vi "pid-toolkit-autotuning-design.vi"() -> ()   [LabVIEW 2018, in "pid-toolkit.lvlib"]
uses:
  <vilib>/Platform/TimedLoop/XDataNode/timing_clust.ctl
  <vilib>/Platform/TimedLoop/XDataNode/nitl_modes.ctl
  <vilib>/Platform/TimedLoop/XDataNode/wakeup.ctl
  <vilib>/addons/control/pid/autopid.llb/PID Autotuning Design (Ziegler-Nichols).vi
  <vilib>/addons/control/pid/autopid.llb/PID Autotuning Design (Cohen-Coon).vi
  <vilib>/addons/control/pid/autopid.llb/PID Autotuning Design (Chien-Hrones-Reswick).vi
  <vilib>/addons/control/pid/autopid.llb/PID Autotuning Design (Internal Model Control).vi
  <vilib>/platform/TimedLoop/XDataNode/XDataNode.xnode
  pid-toolkit.lvlib
  <vilib>/Platform/TimedLoop/XDataNode/XDNodeRunTimeDep.lvlib
  <vilib>/addons/control/pid/NI_PID_autopid.lvlib
panel:
  in  "Tuning specifications":u16(ring) items=["Regulator - 0 %", "Regulator -  20%", "Servo - 0%", "Servo - 20%"]
  in  "Desired Time Constant (tau_c)":dbl
  out "Single Update (Multiple Plots, stacked)":cluster{"Temperature":sgl, "Setpoint":sgl, sgl}(graph)
  out "Output":u16
  out "High":bool
  out "Low":bool
  in  "Manual":u8(slide) scale=0.0..255.0
  out "Stimulus":dbl
  out "Response":dbl
  out "Plant Parameters":T1
  out "PID gains":T2
  in  "Controller Gain (K)":dbl
  in  "Closed Loop":bool
  in  "Ziegler-Nichols Speed":u16(ring) items=["Fast", "Normal", "Slow"]
  out "size(s)":i32
  in  "Method":T3(ring)
  in  "Type of Controller":u16(ring) items=["P", "PI", "PID"]
  out "Modbus error":errorcluster
  in  "Off Hook":bool
  in  "Update Rate":dbl caption="Rate"
  out "Failure":bool
  out "Updating":bool
  in  "Update Now":bool
  in  "Maximum":sgl
  in  "Minimum":sgl
  out "Thermometer":sgl(slide) scale=0.0..260.0
  in  "Force exit out of loop":bool
  out "Interval":i64
  out "Duration":i64
  out "Cycle":i32
  in  "Frequency":dbl(slide) scale=0.1..10.0
  # "Loop"
  # "Modbus"
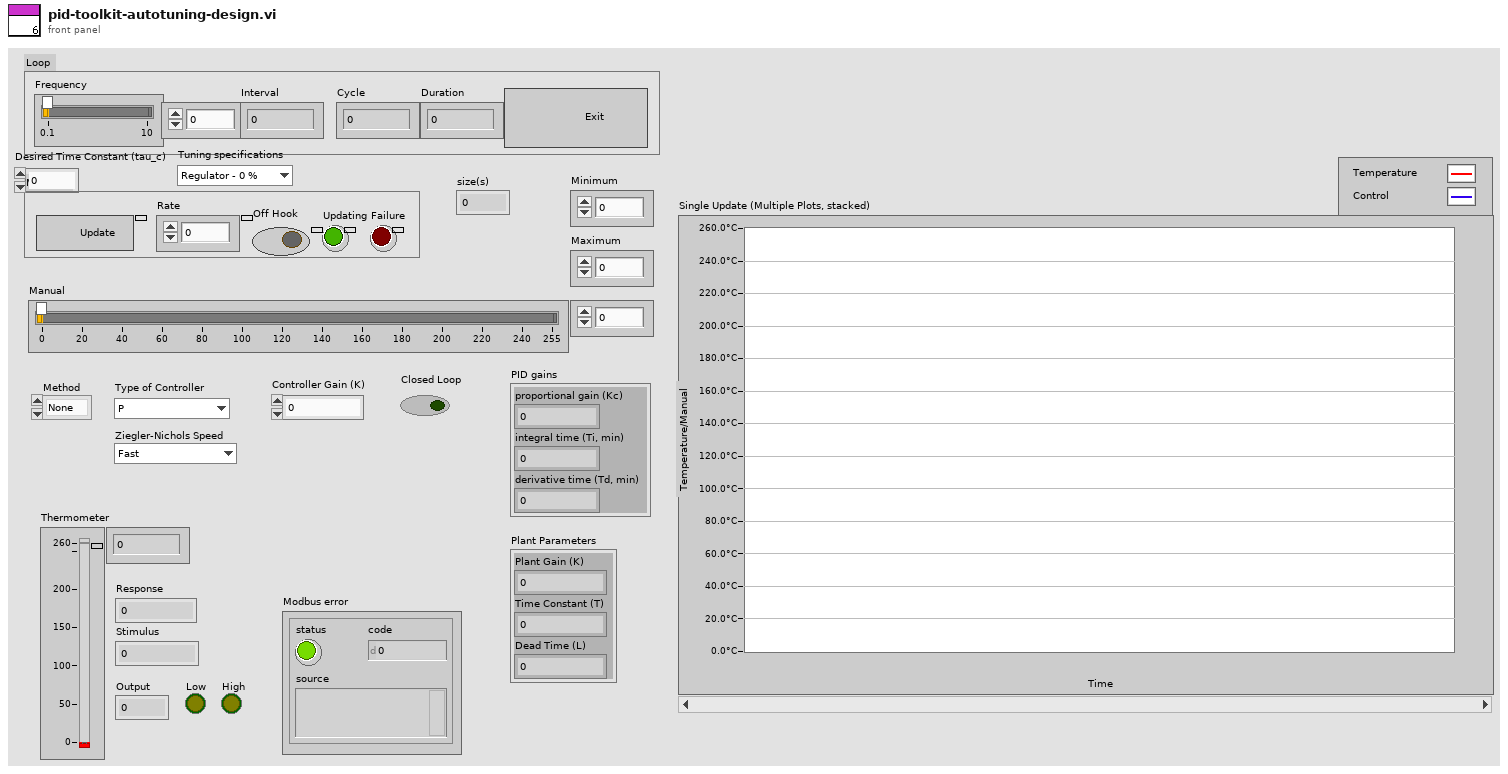
[diagram p1: front panel]
types:
  T1 = cluster{"Plant Gain (K)":dbl, "Time Constant (T)":dbl, "Dead Time (L)":dbl}
  T2 = cluster{"proportional gain (Kc)":dbl, "integral time (Ti, min)":dbl, "derivative time (Td, min)":dbl}
  T3 = enum16{"None", "Ziegler-Nichols", "Cohen-Coon", "Chien-Hrones-Reswick", "Internal Model Control"}
  T4 = typedef "XDNodeRunTimeDep.lvlib/timing_clust.ctl" = cluster{"Expected End [f-1]":u64, "Actual End [f-1]":u64, "Finished Late? [f-1]":bool, "Expected End [i-1]":u64, "Actual End [i-1]":u64, "Finished Late? [i-1]":bool, "Expected Start [i]":u64, "Actual Start [i]":u64, "Expected Start [f]":u64, "Actual Start [f]":u64, "Source Name":string, "Structure Name":string, "Period":i64, "Deadline":i64, "Offset":i64, "Start":i64, "Priority":i32, "Timeout":i32, "Mode":T5, "Wakeup Reason":T6, "Error":errorcluster, "Source Type":string, "Secondary Source Type":string, "Global End Time":u64, "Global Start Time":u64, "Frame Duration":u64, "Iteration Duration":u64, "Assigned CPU":i32, "I/O Scan Engine Mode":u32}
  T5 = typedef "XDNodeRunTimeDep.lvlib/nitl_modes.ctl" = enum32{"No Change", "Process missed periods, maintain original phase", "Discard missed periods, maintain original phase", "Process missed periods, ignore original phase", "Discard missed periods, ignore original phase"}
  T6 = typedef "XDNodeRunTimeDep.lvlib/wakeup.ctl" = enum32{"Normal", "Aborted", "Asynchronous wakeup", "Timing source error", "Timed loop error", "Timeout"}
  T7 = enum8{"Enabled", "Disabled", "Disabled and Grayed Out"}
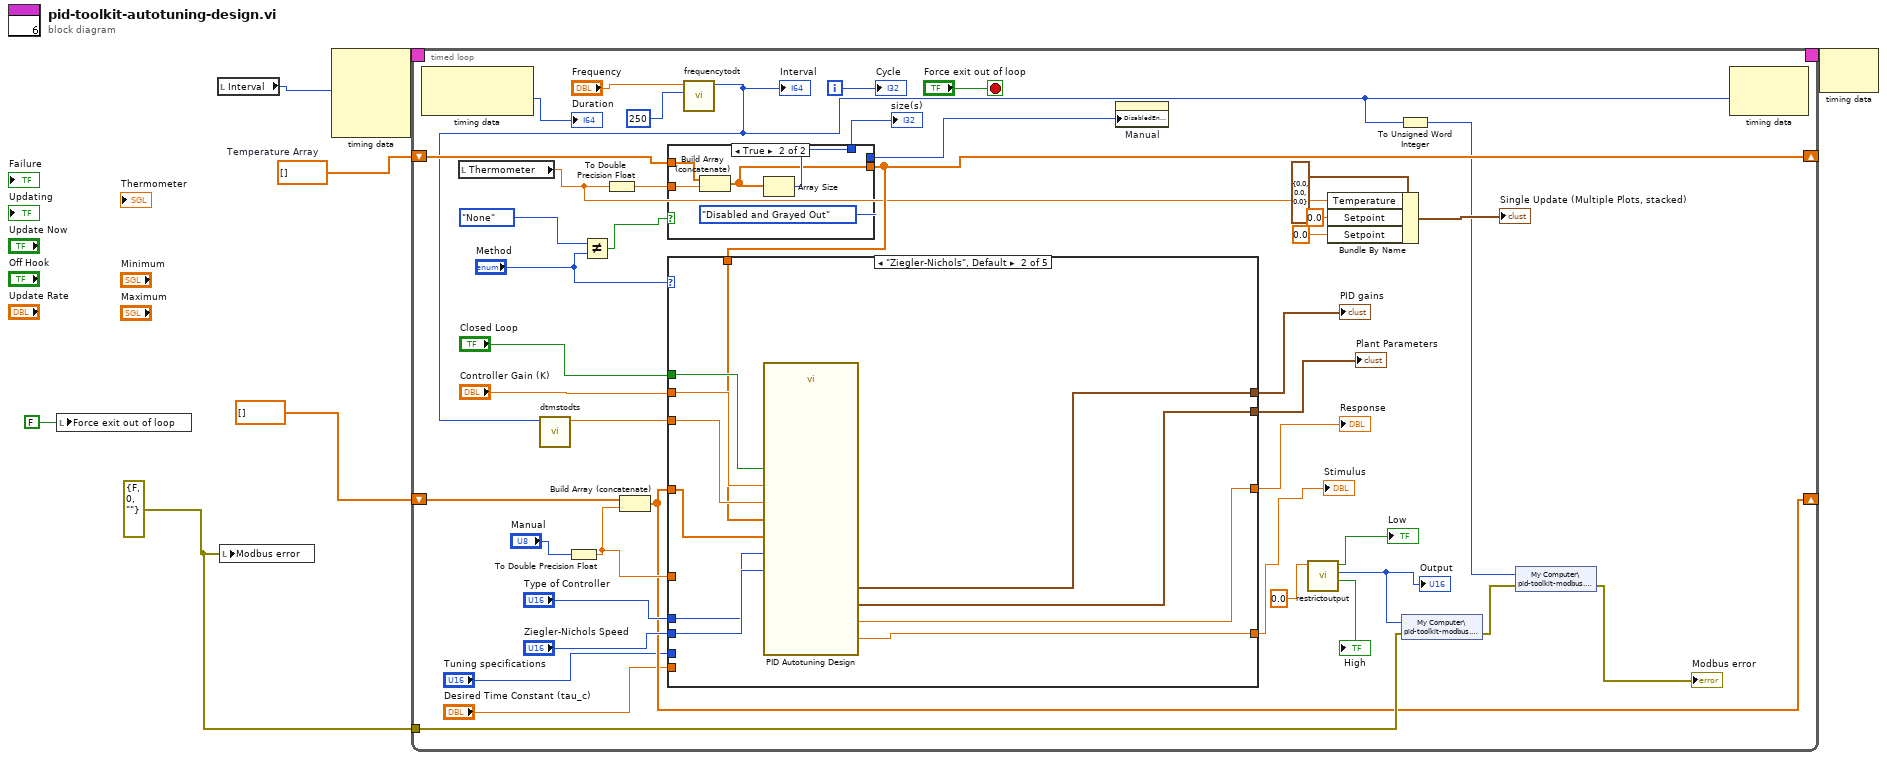
[diagram p0: block diagram]
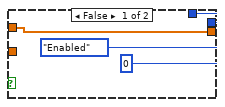
[diagram p2: hidden frame]
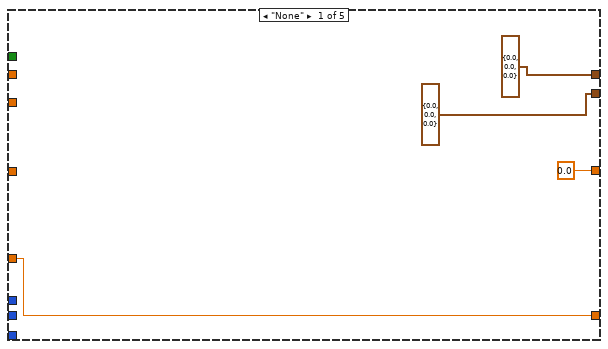
[diagram p3: hidden frame]
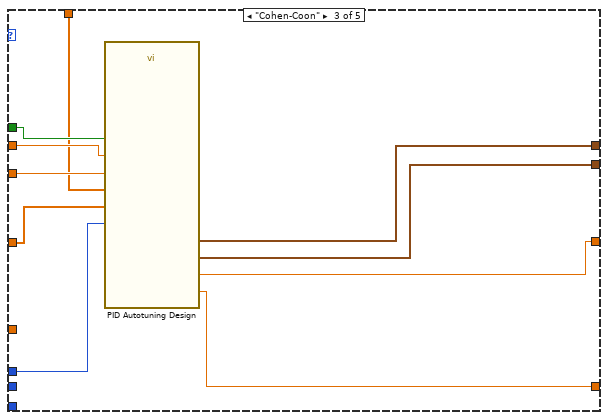
[diagram p4: hidden frame]
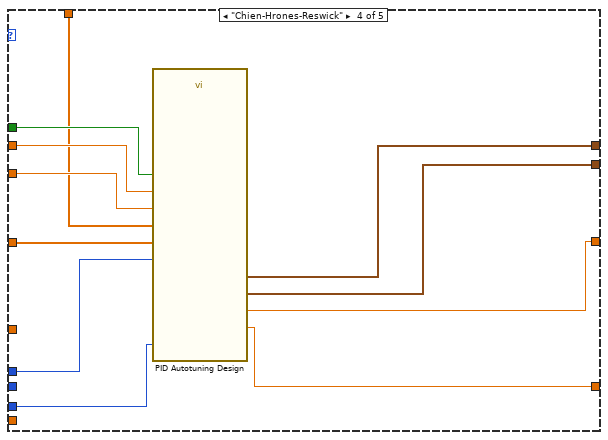
[diagram p5: hidden frame]
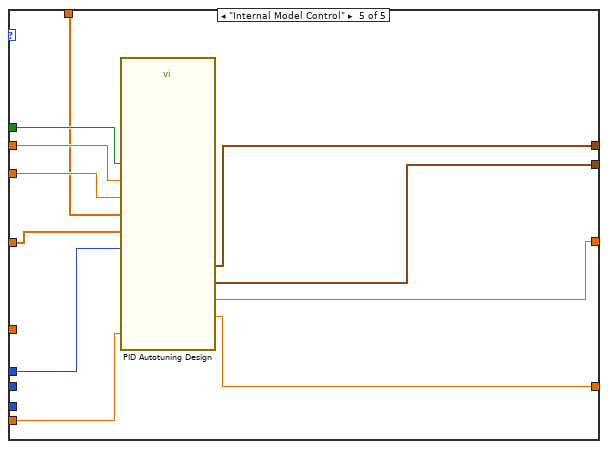
[diagram p6: hidden frame]
diagram:
  w1 = errorcluster {"status"=FALSE, "code"=0, "source"=""} ("Modbus error")
  w4 = dbl[] []  # Temperature Array
  n1 = local write "Force exit out of loop"(FALSE ("Force exit out of loop")) -> ()
  n2 = local read "Interval"() -> (w2:i64)
  n3 = local write "Modbus error"(w1) -> ()
  n4 = node-c288(w2) -> (w7:T4)  [unwired: 3 in]
  n5 = timed-loop {
    timing: w7 -> [_]
    timing-out: [_] -> w6
    shift-right: [w25] -> _
    shift-left: w4 -> [w35]
    shift-right: [w11] -> _
    shift-left: dbl[] [] ("Array") -> [w13]
    tunnel: w1 -> [w32]
    i -> [w45]
    stop <- "Force exit out of loop" stop-if-true
    n6 = node-c288() -> (→"Duration":i64)  [unwired: 1 in, 1 out]
    n7 = local read "Thermometer"() -> (w22:sgl)
    n8 = To Double Precision Float(number="Manual") -> (double precision float=w12:dbl)
    n9 = Not Equal?(x=T3."None" ("Method"), y="Method") -> (x != y?=w27:bool)
    n10 = To Double Precision Float(number=w22) -> (double precision float=w34:dbl)
    n11 = Build Array (concatenate)(w13, w12) -> (w11:dbl[])
    n12 = case shown="True" w27 {
      tunnel: w35 -> [w52 w57]
      tunnel: w34 -> [_ w56]
      tunnel: [0 w55] -> w33
      tunnel: [w52 w54] -> w25
      tunnel: [T7."Enabled" ("Disabled") T7."Disabled and Grayed Out" ("Disabled")] -> w30
      frame False {
      }
      frame True {
        n13 = Build Array (concatenate)(w57, w56) -> (w54:dbl[])
        n14 = Array Size(array=w54) -> (size(s)=w55:i32)
      }
    }
    "size(s)" <- w33
    n15 = call "frequencytodt.vi"("Default in"=i64 250, "Frequency"="Frequency") -> ("Default out"=w16:i64)  [unwired: 9 in]
    "Interval" <- w16
    n16 = call "dtmstodts.vi"("Default in"=w16) -> ("Numeric"=w43:dbl)  [unwired: 10 in]
    n17 = case shown="\"Ziegler-Nichols\", Default" "Method" {
      tunnel: "Closed Loop" -> [_ w72 w82 w93 w104]
      tunnel: w43 -> [_ w70 w80 w91 w102]
      tunnel: "Controller Gain (K)" -> [_ w71 w81 w92 w103]
      tunnel: [T2 {"proportional gain (Kc)"=0.0, "integral time (Ti, min)"=0.0, "derivative time (Td, min)"=0.0} ("PID gains") w69 w77 w89 w99] -> w41
      tunnel: [T1 {"Plant Gain (K)"=0.0, "Time Constant (T)"=0.0, "Dead Time (L)"=0.0} ("Plant Parameters") w68 w76 w88 w98] -> w40
      tunnel: [0.0 ("response operating point") w67 w75 w87 w97] -> w39
      tunnel: [w58 w66 w74 w86 w96] -> w15
      tunnel: "Ziegler-Nichols Speed" -> [_ w65 _ _ _]
      tunnel: "Type of Controller" -> [_ w64 w79 w85 w100]
      tunnel: w25 -> [_ w63 w78 w90 w101]
      tunnel: w12 -> [w58 _ _ _ _]
      tunnel: w11 -> [_ w62 w73 w84 w94]
      tunnel: "Desired Time Constant (tau_c)" -> [_ _ _ _ w95]
      tunnel: "Tuning specifications" -> [_ _ _ w83 _]
      frame "None" {
      }
      frame "Ziegler-Nichols", Default {
        n18 = call-poly <vilib>:"PID Autotuning Design.vi"("Ziegler-Nichols Speed"=w65, "Controller Gain (K)"=w71, "Type of Controller"=w64, "dt (s)"=w70, "closed-loop?"=w72, "Response signal"=w63, "Stimulus signal"=w62) -> ("PID gains"=w69:T2, "response operating point"=w67:dbl, "stimulus operating point"=w66:dbl, "Plant Parameters"=w68:T1)  [unwired: 1 in]
      }
      frame "Cohen-Coon" {
        n19 = call-poly <vilib>:"PID Autotuning Design.vi"("Controller Gain (K)"=w81, "Type of Controller"=w79, "dt (s)"=w80, "closed-loop?"=w82, "Response signal"=w78, "Stimulus signal"=w73) -> ("PID gains"=w77:T2, "response offset"=w75:dbl, "stimulus offset"=w74:dbl, "Plant Parameters"=w76:T1)  [unwired: 2 in]
      }
      frame "Chien-Hrones-Reswick" {
        n20 = call-poly <vilib>:"PID Autotuning Design.vi"("Tuning specifications"=w83, "Controller Gain (K)"=w92, "Type of Controller"=w85, "dt (s)"=w91, "closed-loop?"=w93, "Response signal"=w90, "Stimulus signal"=w84) -> ("PID gains"=w89:T2, "response offset"=w87:dbl, "stimulus offset"=w86:dbl, "Plant Parameters"=w88:T1)  [unwired: 1 in]
      }
      frame "Internal Model Control" {
        n21 = call-poly <vilib>:"PID Autotuning Design.vi"("Desired Time Constant (tau_c)"=w95, "Controller Gain (K)"=w103, "Type of Controller"=w100, "dt (s)"=w102, "closed-loop?"=w104, "Response signal"=w101, "Stimulus signal"=w94) -> ("PID gains"=w99:T2, "response offset"=w97:dbl, "stimulus offset"=w96:dbl, "Plant Parameters"=w98:T1)  [unwired: 1 in]
      }
    }
    "PID gains" <- w41
    "Plant Parameters" <- w40
    "Response" <- w39
    "Stimulus" <- w15
    n22 = property on="Manual" class="Slide (strict)"("DisabledEnum"=w30) -> ()  [unwired: 2 in, 2 out]
    n23 = call "restrictoutput.vi"("Input"=0.0) -> ("Hig"=→"High":bool, "Output"=w26:u16, "Low"=→"Low":bool)  [unwired: 8 in]
    "Output" <- w26
    n24 = Bundle By Name(cluster=cluster{"Temperature":sgl, "Setpoint":sgl, sgl} {"Temperature"=0.0, "Setpoint"=0.0, 0.0} ("Single Update (Multiple Plots, stacked)"), "Temperature"=w22, "Setpoint"=sgl 0.0, "Setpoint"=sgl 0.0) -> (→"Single Update (Multiple Plots, stacked)":cluster{"Temperature":sgl, "Setpoint":sgl, sgl})
    n25 = To Unsigned Word Integer(number=w16) -> (unsigned 16bit integer=w17:u16)
    n26 = shared-variable "My Computer\\pid-toolkit-modbus.lvlib\\400002"(w26, error in=w32) -> (error out=w19:errorcluster)
    n27 = shared-variable "My Computer\\pid-toolkit-modbus.lvlib\\400001"(w17, error in=w19) -> (error out=→"Modbus error":errorcluster)
    n28 = node-c288(w16) -> ()  [unwired: 1 in, 1 out]
    "Cycle" <- w45
  }
  n29 = node-c288(w6) -> ()  [unwired: 1 out]
